vi "zadanie_2_haslo.vi"() -> ()   [LabVIEW 2024]
panel:
  out "valid?":bool
  in  "password":string
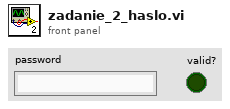
[diagram p1: front panel]
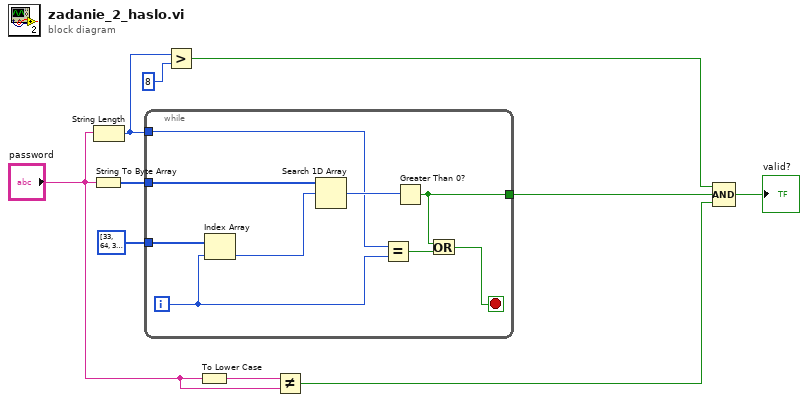
[diagram p0: block diagram]
diagram:
  n1 = String To Byte Array(string="password") -> (unsigned byte array=w9:u8[])
  n2 = String Length(string="password") -> (length=w4:i32)
  n3 = while {
    tunnel: w9 -> [w19]
    tunnel: u8[] [33, 64, 35, 36, 37, 38, 42, 40, 41] ("Array") -> [w18]
    tunnel: [w14] -> w6
    tunnel: w4 -> [w12]
    i -> [w13]
    stop <- w15 stop-if-true
    n4 = Index Array(array=w18, index=w13) -> (element=w17:u8)
    n5 = Search 1D Array(1D array=w19, element=w17) -> (index of element=w16:i32)  [unwired: 1 in]
    n6 = Equal?(x=w12, y=w13) -> (x = y?=w11:bool)
    n7 = Greater Than 0?(x=w16) -> (x > 0?=w14:bool)
    n8 = Or(x=w14, y=w11) -> (x .or. y?=w15:bool)
  }
  n9 = Greater?(x=w4, y=8) -> (0:w5:bool)
  n10 = To Lower Case(string="password") -> (all lower case string=w3:string)
  n11 = Not Equal?(x=w3, y="password") -> (x != y?=w1:bool)
  n12 = Compound Arithmetic op=AND(w5, w6, w1) -> (→"valid?":bool)
